vi "induction-furnace-control.vi"() -> ()   [LabVIEW 2019]
uses:
  <vilib>/DAQmx/read.llb/DAQmx Read (Analog 1D DBL 1Chan NSamp).vi
  <vilib>/Analysis/baseanly.llb/Mean (DBL).vi
  <vilib>/DAQmx/write.llb/DAQmx Write (Analog DBL 1Chan 1Samp).vi
  <vilib>/addons/control/pid/pid.llb/PID (DBL).vi
  <vilib>/DAQmx/create/channels.llb/DAQmx Create Channel (AO-Current-Basic).vi
  <vilib>/DAQmx/create/channels.llb/DAQmx Create Channel (AI-Current-Basic).vi
  <vilib>/DAQmx/miscellaneous.llb/DAQmx Fill In Error Info.vi
  <vilib>/addons/control/pid/NI_PID_pid.lvlib
  <vilib>/Analysis/NI_AALBase.lvlib
panel:
  out "VALVE OUTPUT":dbl
  in  "ENABLE FURNACE":bool[](array[boolean])
  in  "STOP FURNACE":bool[](array[boolean])
  in  "CLOSE VALVE":bool[](array[boolean])
  in  "PURGE FLOW":bool[](array[boolean])
  in  "Emergency":bool
  in  "ESTOP":bool
  in  "POWER OUT":dbl format="%#_13g"
  out "PYROMETER TEMP":dbl
  out "DONE":bool
  in  "ARGON OUT":dbl format="%#_13g"
  in  "MAIN STATE":T1(ring)
  out "MAIN PAGES":T2(tab)
  in  "TEST SETTINGS":bool
  in  "START TEST CYCLE":bool
  in  "START ARGON PURGE CYCLE":bool
  out "TIME TILL PURGE CYCLE FINISHES":dbl
  in  "START HEATING CYCLE":bool
  out "CURRENT RAMP UP POWER LEVEL":string
  out "PYROMETER TEMP RAMP UP":dbl
  out "FINAL TEMPERATURE GOAL (C)":dbl
  out "CURRENT SET POINT (C)":dbl
  out "CURRENT TEMPERATURE (C)":dbl
  out "POWER LEVEL OUTPUT (%)":dbl
  out "TEMPERATURE OVER TIME":cluster{dbl[], dbl[]}[](graph)
  out "CURRENT RAMP DOWN POWER LEVEL":string
  in  "END PROGRAM":bool
  in  "RESET PROGRAM":bool
  in  "GO BACK":bool
  in  "HOLD TIME (min)":dbl
  in  "PURGE TIMER TIME (min)":dbl
  in  "PID FINAL TEMP (C)":dbl
  in  "PID CONTROL START TEMP (C)":dbl=850.0
  in  "SAVE SETTINGS":bool
  # "Once you have loaded your sample, drawn a high vacuum, and are ready to start your test press the button below"
  # "Once you have started the purge cycle on the vacuum pump, press the button below to start the argon purge flow."
  # "min"
  # "Once you are ready to start heating up the sample, press the button below"
  # "CYCLE IS NOW FINISHED, PLEASE UNPLUG THE MASS FLOW METER.\nIF YOU WANT TO START ANOTHER TEST PRESS THE RESET BUTTON BELOW. IF NOT PRESS END."
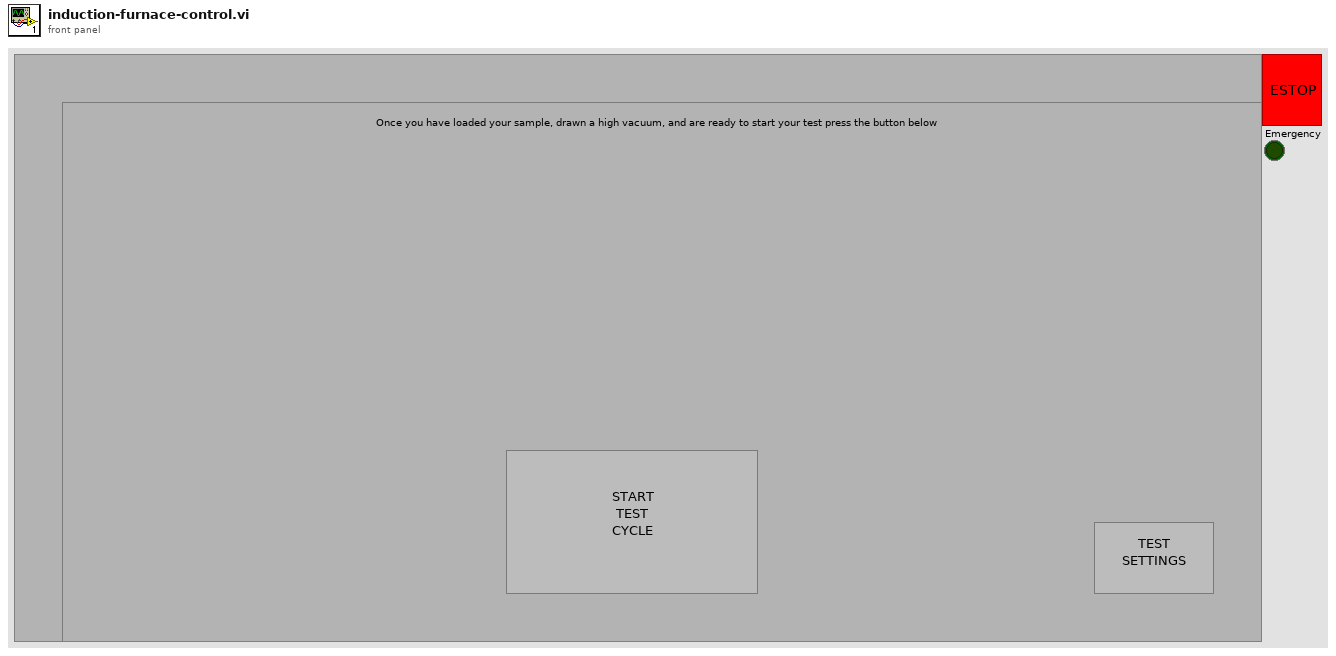
[diagram p1: front panel]
types:
  T1 = enum16{"INIT", "IDLE", "START CYCLE", "START ARGON PURGE", "ARGON TIMER", "START ARGON FLOW", "START HEATING CYCLE", "RAMP UP", "PID CONTROL", "HOLD", "PID DOWN", "RAMP DOWN", "END"}
  T2 = enum32{"START CYCLE", "START ARGON PURGE", "PURGE TIMER", "START HEATING CYCLE", "RAMP UP", "PID", "RAMP DOWN", "CYCLE FINISHED", "SETTINGS"}
  T3 = cluster{"proportional gain (Kc)":dbl, "integral time (Ti, min)":dbl, "derivative time (Td, min)":dbl}
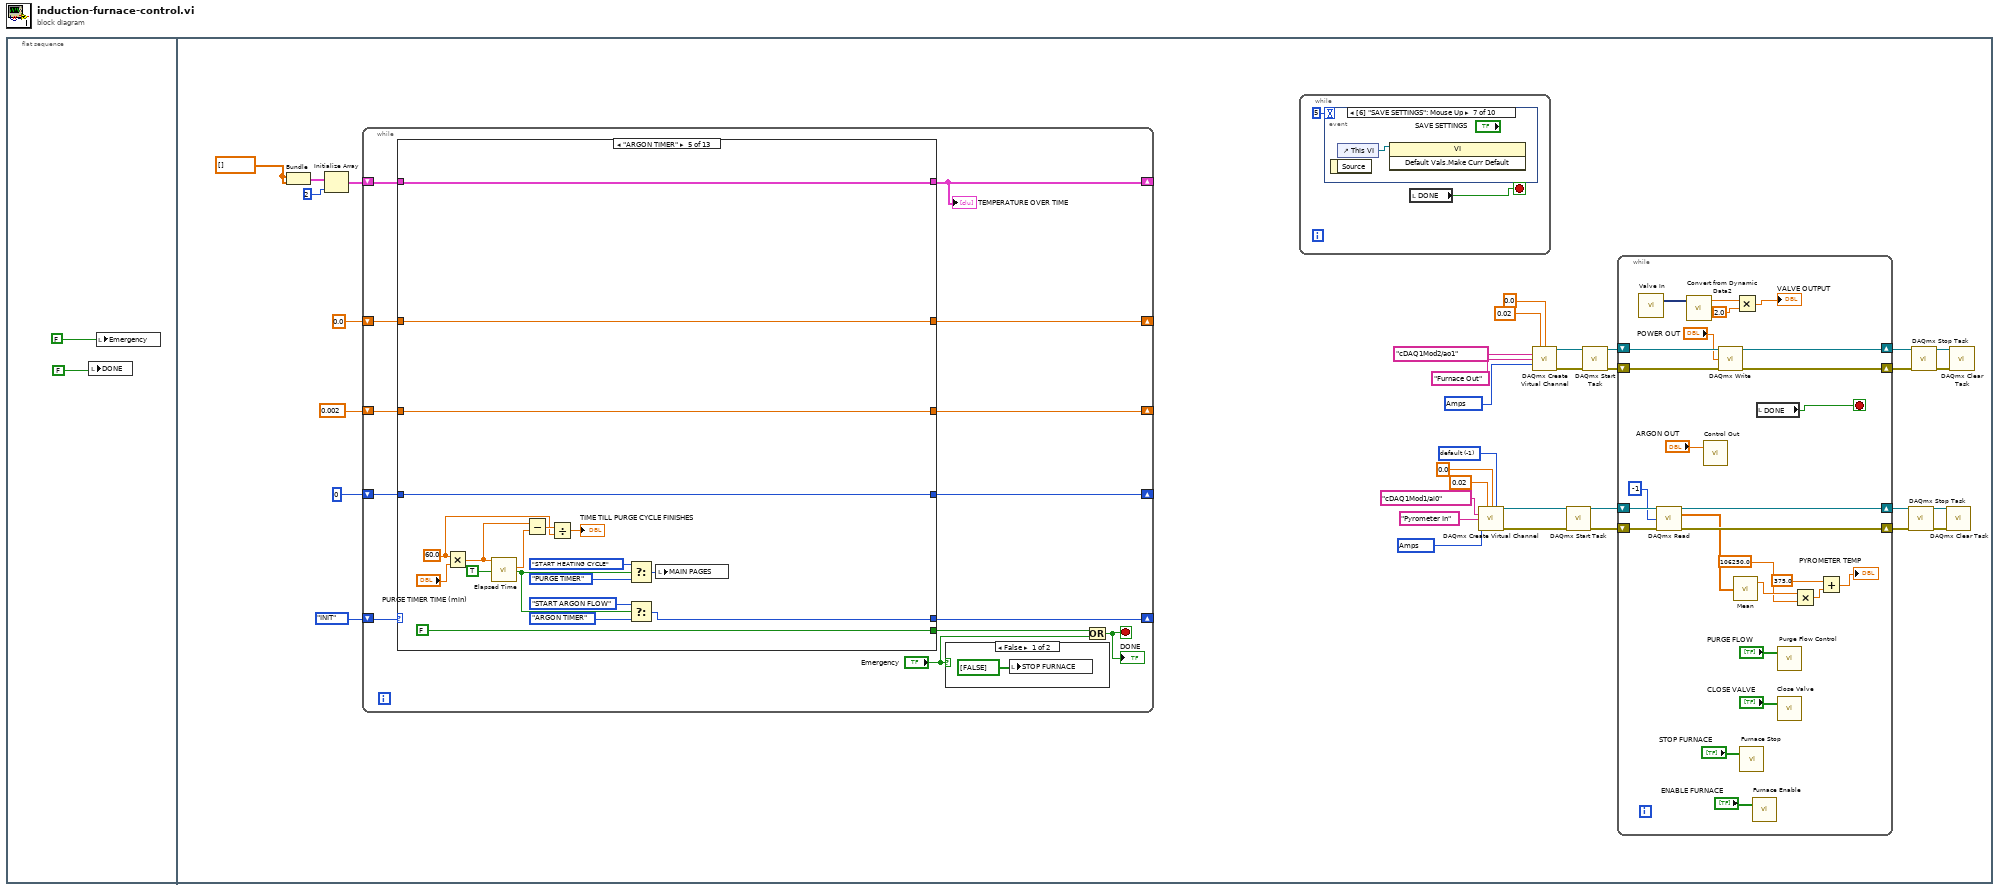
[diagram p0: block diagram]
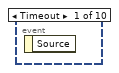
[diagram p2: hidden frame]
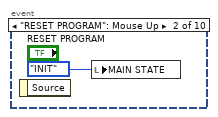
[diagram p3: hidden frame]
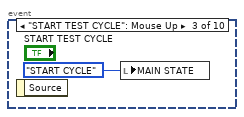
[diagram p4: hidden frame]
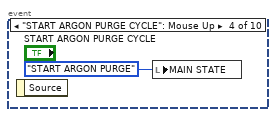
[diagram p5: hidden frame]
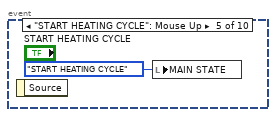
[diagram p6: hidden frame]
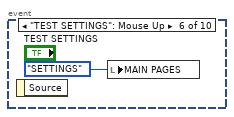
[diagram p7: hidden frame]
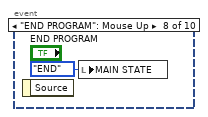
[diagram p8: hidden frame]
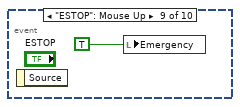
[diagram p9: hidden frame]
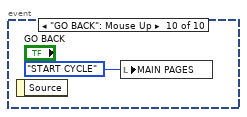
[diagram p10: hidden frame]
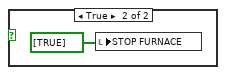
[diagram p11: hidden frame]
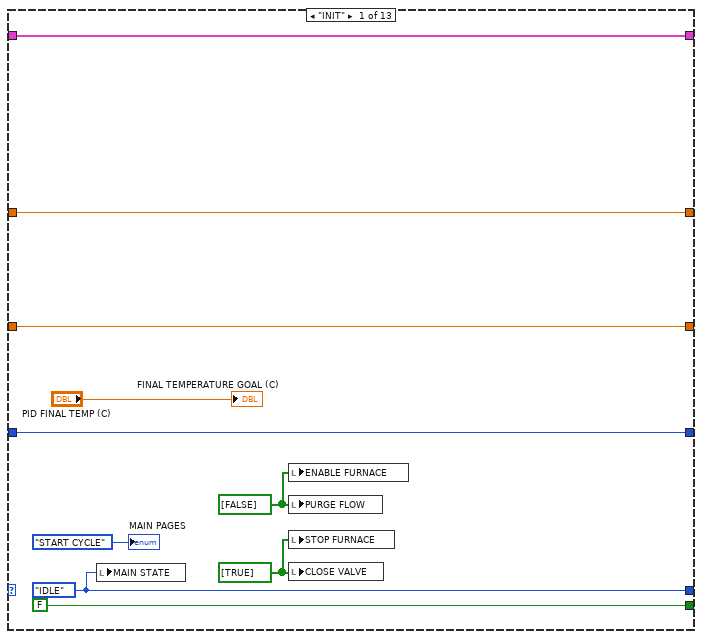
[diagram p12: hidden frame]
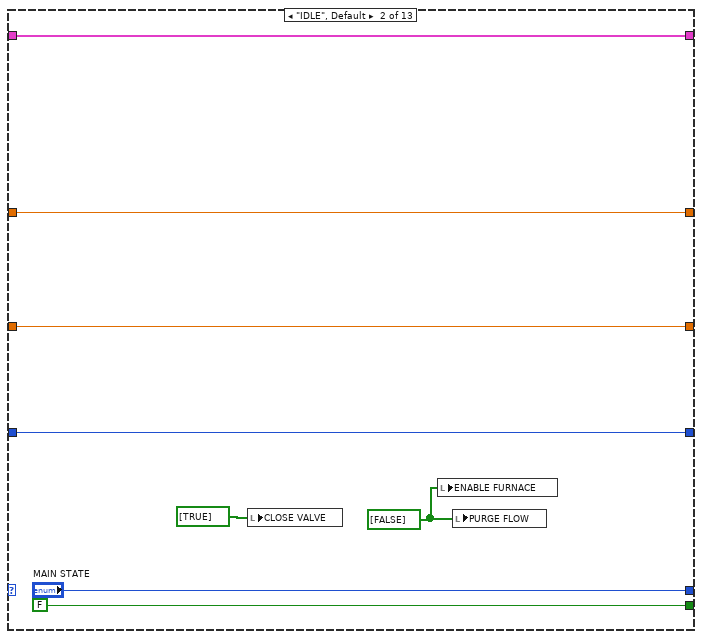
[diagram p13: hidden frame]
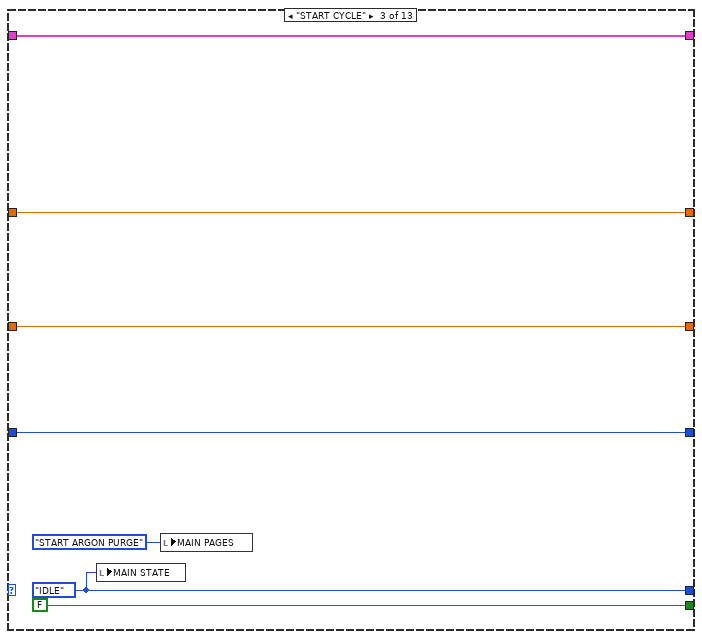
[diagram p14: hidden frame]
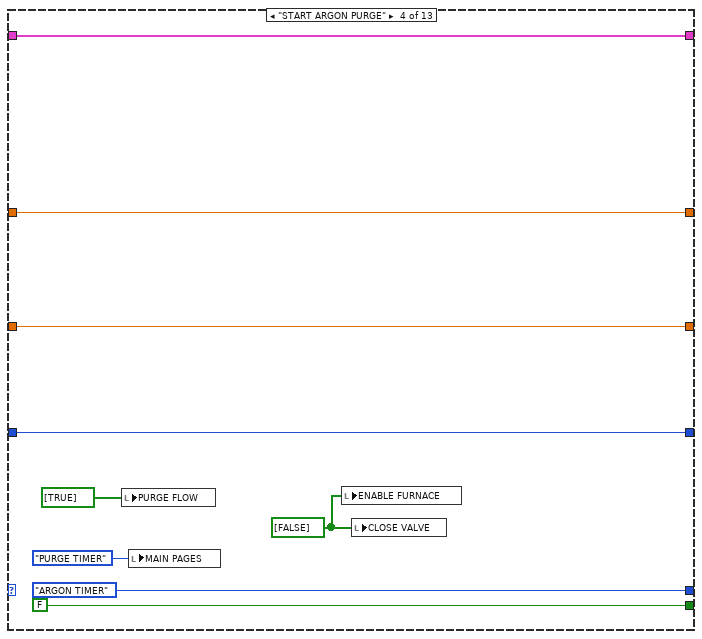
[diagram p15: hidden frame]
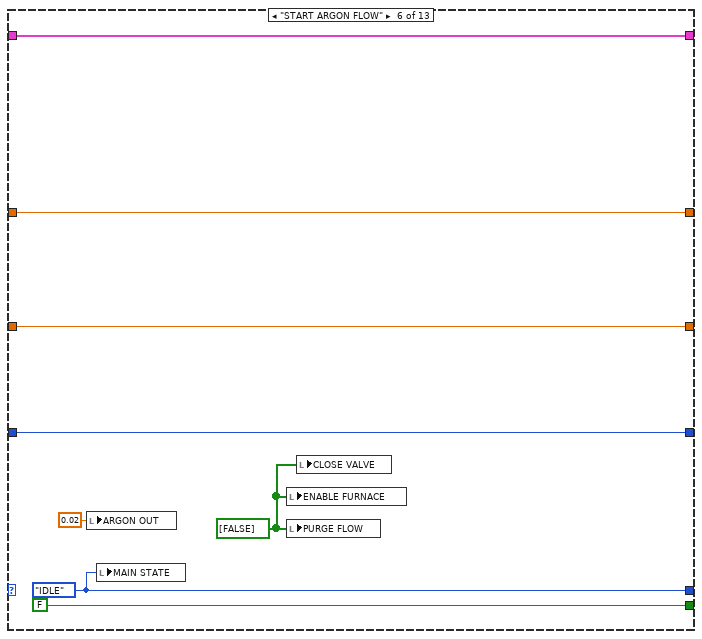
[diagram p16: hidden frame]
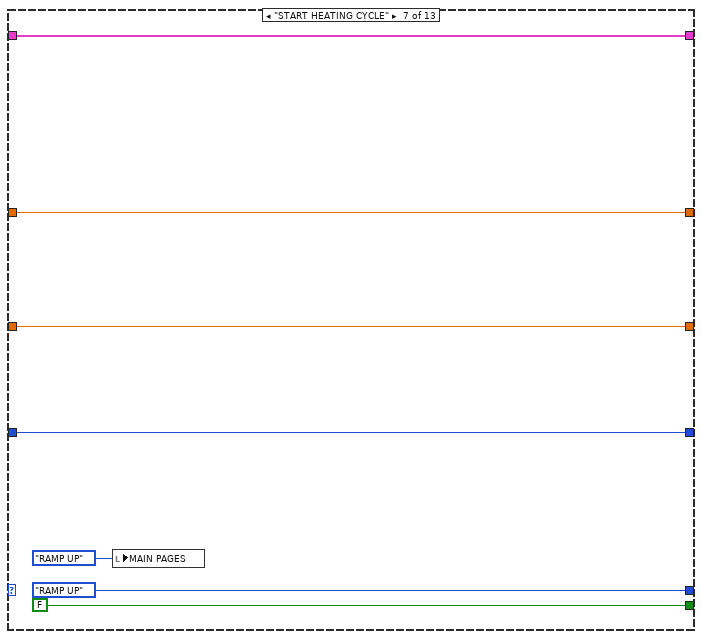
[diagram p17: hidden frame]
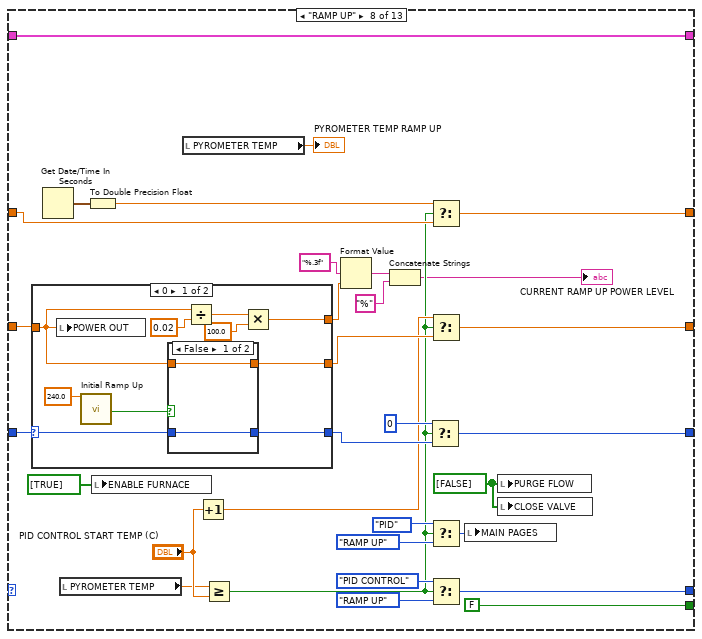
[diagram p18: hidden frame]
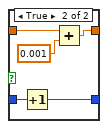
[diagram p19: hidden frame]
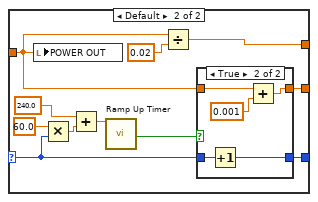
[diagram p20: hidden frame]
diagram:
  n1 = flat-sequence {
    frame #0 {
      n2 = local write "DONE"(FALSE) -> ()
      n3 = local write "Emergency"(FALSE) -> ()
    }
    frame #1 {
      w11 = -1 items=["default"=-1, "RSE"=10083, "NRSE"=10078, "Differential"=10106, "Pseudodifferential"=12529] ("input terminal configuration")
      w12 = 10342 items=["Amps"=10342, "From Custom Scale"=10065] ("units")
      w17 = 10342 items=["Amps"=10342, "From Custom Scale"=10065] ("units")
      w34 = dbl[] []
      n4 = Bundle(w34, w34) -> (w36:cluster{dbl[], dbl[]})  [unwired: 1 in]
      n5 = Initialize Array(w36, 2 ("dimension size")) -> (w33:cluster{dbl[], dbl[]}[])
      n6 = while {
        shift-right: [w86] -> _
        shift-left: T1."INIT" -> [w87]
        shift-right: [w76] -> _
        shift-left: w33 -> [w83]
        shift-right: [w81] -> _
        shift-left: 0.002 ("Ramp Power") -> [w82]
        shift-right: [w79] -> _
        shift-left: 0 ("Ramp Up Counter") -> [w80]
        shift-right: [w77] -> _
        shift-left: 0.0 ("PID Start Time") -> [w78]
        stop <- w84 stop-if-true
        n7 = case shown="\"ARGON TIMER\"" w87 {
          tunnel: [w99 "MAIN STATE" w112 T1."ARGON TIMER" ("MAIN STATE") w133 w148 T1."RAMP UP" w183 w246 w271 w315 w381 T1."END" ("MAIN STATE")] -> w86
          tunnel: [FALSE FALSE FALSE FALSE FALSE FALSE FALSE FALSE FALSE FALSE FALSE FALSE TRUE] -> w85
          tunnel: w83 -> [w94 w105 w111 w119 w128 w147 w154 w180 w239 w292 w322 w377 w396]
          tunnel: [w94 w105 w111 w119 w128 w147 w154 w180 w225 w291 w319 w377 w396] -> w76
          tunnel: w82 -> [w92 w104 w110 w117 w126 w146 w153 w178 w256 w276 w345 w376 w392]
          tunnel: [w92 w104 w110 w117 w126 w146 w153 w171 w229 w276 w311 w366 w392] -> w81
          tunnel: w80 -> [w91 w103 w109 w118 w125 w145 w152 w176 w224 w277 w318 w371 w391]
          tunnel: [w91 w103 w109 w118 w125 w145 w152 w174 w224 w277 w318 w371 w391] -> w79
          tunnel: w78 -> [w90 w102 w108 w116 w124 w144 w151 w167 w242 w290 w321 w365 _]
          tunnel: [w90 w102 w108 w116 w124 w144 w151 w164 w242 w290 w321 w365 0.0 ("PID Start Time")] -> w77
          frame "INIT" {
            w95 = bool[] [FALSE] ("CLOSE VALVE")
            w96 = bool[] [TRUE] ("CLOSE VALVE")
            w99 = T1."IDLE" ("MAIN STATE")
            n8 = local write "MAIN STATE"(w99) -> ()
            n9 = local write "ENABLE FURNACE"(w95) -> ()
            n10 = local write "PURGE FLOW"(w95) -> ()
            n11 = local write "STOP FURNACE"(w96) -> ()
            n12 = local write "CLOSE VALVE"(w96) -> ()
            "MAIN PAGES" <- T2."START CYCLE" ("MAIN PAGES")
            "FINAL TEMPERATURE GOAL (C)" <- "PID FINAL TEMP (C)"
          }
          frame "IDLE", Default {
            w100 = bool[] [FALSE] ("CLOSE VALVE")
            n13 = local write "CLOSE VALVE"(bool[] [TRUE] ("CLOSE VALVE")) -> ()
            n14 = local write "ENABLE FURNACE"(w100) -> ()
            n15 = local write "PURGE FLOW"(w100) -> ()
          }
          frame "START CYCLE" {
            w112 = T1."IDLE" ("MAIN STATE")
            n16 = local write "MAIN STATE"(w112) -> ()
            n17 = local write "MAIN PAGES"(T2."START ARGON PURGE" ("MAIN PAGES")) -> ()
          }
          frame "START ARGON PURGE" {
            w115 = bool[] [FALSE] ("CLOSE VALVE")
            n18 = local write "PURGE FLOW"(bool[] [TRUE] ("CLOSE VALVE")) -> ()
            n19 = local write "MAIN PAGES"(T2."PURGE TIMER" ("MAIN PAGES")) -> ()
            n20 = local write "ENABLE FURNACE"(w115) -> ()
            n21 = local write "CLOSE VALVE"(w115) -> ()
          }
          frame "ARGON TIMER" {
            w138 = 60.0 ("y")
            n22 = Multiply(x=w138, y="PURGE TIMER TIME (min)") -> (x*y=w142:dbl)
            n23 = call "Elapsed Time"("Time Target (s)"=w142, "Auto Reset"=TRUE ("Reset")) -> ("Elapsed Time (s)"=w141:dbl, "Time has Elapsed"=w132:bool)  [unwired: 10 in, 6 out]
            n24 = Subtract(x=w142, y=w141) -> (x-y=w139:dbl)
            n25 = Divide(x=w139, y=w138) -> (x/y=→"TIME TILL PURGE CYCLE FINISHES":dbl)
            n26 = Select(t=T2."START HEATING CYCLE" ("MAIN PAGES"), s=w132, f=T2."PURGE TIMER" ("MAIN PAGES")) -> (s? t:f=w131:T2)
            n27 = Select(t=T1."START ARGON FLOW", s=w132, f=T1."ARGON TIMER") -> (s? t:f=w133:T1)
            n28 = local write "MAIN PAGES"(w131) -> ()
          }
          frame "START ARGON FLOW" {
            w143 = bool[] [FALSE] ("CLOSE VALVE")
            w148 = T1."IDLE" ("MAIN STATE")
            n29 = local write "ARGON OUT"(0.02 ("CONTROL OUT")) -> ()
            n30 = local write "MAIN STATE"(w148) -> ()
            n31 = local write "ENABLE FURNACE"(w143) -> ()
            n32 = local write "PURGE FLOW"(w143) -> ()
            n33 = local write "CLOSE VALVE"(w143) -> ()
          }
          frame "START HEATING CYCLE" {
            n34 = local write "MAIN PAGES"(T2."RAMP UP" ("MAIN PAGES")) -> ()
          }
          frame "RAMP UP" {
            w182 = bool[] [FALSE] ("CLOSE VALVE")
            n35 = case shown="0" w176 {
              selector: w176 -> [w196 w208]
              tunnel: [w190 w214] -> w177
              tunnel: w178 -> [w195 w213]
              tunnel: [w193 w207] -> w172
              tunnel: [w192 w206] -> w173
              frame 0 {
                n36 = local write "POWER OUT"(w195) -> ()
                n37 = call "Initial Ramp Up"("Time Target (s)"=240.0) -> ("Time has Elapsed"=w198:bool)  [unwired: 11 in, 7 out]
                n38 = case shown="False" w198 {
                  tunnel: w196 -> [w199 w205]
                  tunnel: w195 -> [w200 w204]
                  tunnel: [w200 w202] -> w193
                  tunnel: [w199 w201] -> w192
                  frame False {
                  }
                  frame True {
                    n39 = Increment(x=w205) -> (x+1=w201:i32)
                    n40 = Add(x=w204, y=0.001) -> (x+y=w202:dbl)
                  }
                }
                n41 = Divide(x=w195, y=0.02) -> (x/y=w191:dbl)
                n42 = Multiply(x=w191, y=100.0) -> (x*y=w190:dbl)
              }
              frame Default {
                n43 = local write "POWER OUT"(w213) -> ()
                n44 = Multiply(x=60.0 ("Time Target (s)"), y=w208) -> (x*y=w211:dbl)
                n45 = Add(x=240.0 ("Time Target (s)"), y=w211) -> (x+y=w210:dbl)
                n46 = call "Ramp Up Timer"("Time Target (s)"=w210) -> ("Time has Elapsed"=w216:bool)  [unwired: 11 in, 7 out]
                n47 = Divide(x=w213, y=0.02) -> (x/y=w214:dbl)
                n48 = case shown="True" w216 {
                  tunnel: w208 -> [w218 w223]
                  tunnel: w213 -> [w217 w222]
                  tunnel: [w217 w220] -> w207
                  tunnel: [w218 w219] -> w206
                  frame False {
                  }
                  frame True {
                    n49 = Increment(x=w223) -> (x+1=w219:i32)
                    n50 = Add(x=w222, y=0.001) -> (x+y=w220:dbl)
                  }
                }
              }
            }
            n51 = Get Date/Time In Seconds() -> (seconds since 1Jan1904=w170:timestamp)
            n52 = local read "PYROMETER TEMP"() -> (w162:dbl)
            n53 = To Double Precision Float(number=w170) -> (double precision float=w166:dbl)
            n54 = local write "ENABLE FURNACE"(bool[] [TRUE] ("CLOSE VALVE")) -> ()
            n55 = local read "PYROMETER TEMP"() -> (→"PYROMETER TEMP RAMP UP":dbl)
            n56 = Increment(x="PID CONTROL START TEMP (C)") -> (x+1=w169:dbl)
            n57 = Greater Or Equal?(x=w162, y="PID CONTROL START TEMP (C)") -> (x >= y?=w165:bool)
            n58 = Format Value(format string="%.3f", value (0)=w177) -> (output string=w161:string)  [unwired: 1 in]
            n59 = Concatenate Strings(w161, "%" ("format string")) -> (→"CURRENT RAMP UP POWER LEVEL":string)
            n60 = Select(t=0 ("Ramp Up Counter"), s=w165, f=w173) -> (s? t:f=w174:i32)
            n61 = Select(t=w166, s=w165, f=w167) -> (s? t:f=w164:dbl)
            n62 = Select(t=w169, s=w165, f=w172) -> (s? t:f=w171:dbl)
            n63 = Select(t=T2."PID" ("MAIN PAGES"), s=w165, f=T2."RAMP UP" ("MAIN PAGES")) -> (s? t:f=w188:T2)
            n64 = Select(t=T1."PID CONTROL", s=w165, f=T1."RAMP UP") -> (s? t:f=w183:T1)
            n65 = local write "MAIN PAGES"(w188) -> ()
            n66 = local write "PURGE FLOW"(w182) -> ()
            n67 = local write "CLOSE VALVE"(w182) -> ()
          }
          frame "PID CONTROL" {
            w262 = bool[] [FALSE] ("CLOSE VALVE")
            n68 = Get Date/Time In Seconds() -> (seconds since 1Jan1904=w260:timestamp)
            n69 = local read "PID FINAL TEMP (C)"() -> (w245:dbl)
            n70 = call "Rate Delay"("Time Target (s)"=6.0) -> ("Time has Elapsed"=w257:bool)  [unwired: 11 in, 7 out]
            n71 = To Double Precision Float(number=w260) -> (double precision float=w259:dbl)
            n72 = Subtract(x=w259, y=w242) -> (x-y=w235:dbl)
            n73 = local write "MAIN PAGES"(T2."PID" ("MAIN PAGES")) -> ()
            n74 = local write "PURGE FLOW"(w262) -> ()
            n75 = local write "CLOSE VALVE"(w262) -> ()
            n76 = local write "ENABLE FURNACE"(bool[] [TRUE] ("CLOSE VALVE")) -> ()
            n77 = local read "PYROMETER TEMP"() -> (w233:dbl)
            "CURRENT TEMPERATURE (C)" <- w233
            n78 = Index Array(array=w239, index #1=0 ("index"), index #2=1 ("index")) -> (element #1=w238:cluster{dbl[], dbl[]}, element #2=w237:cluster{dbl[], dbl[]})
            n79 = case shown="True" w257 {
              tunnel: w256 -> [w265 w267]
              tunnel: [w265 w268] -> w229
              tunnel: w245 -> [_ w270]
              tunnel: [FALSE w266] -> w244
              frame False {
              }
              frame True {
                n80 = Increment(x=w267) -> (x+1=w269:dbl)
                n81 = Equal?(x=w267, y=w270) -> (x = y?=w266:bool)
                n82 = Select(t=w267, s=w266, f=w269) -> (s? t:f=w268:dbl)
              }
            }
            "CURRENT SET POINT (C)" <- w229
            n83 = Unbundle(w238) -> (w236:dbl[], w232:dbl[])
            n84 = Unbundle(w237) -> (w230:dbl[])  [unwired: 1 out]
            n85 = Select(t=T1."HOLD", s=w244, f=T1."PID CONTROL") -> (s? t:f=w246:T1)
            n86 = Build Array (concatenate)(w236, w235) -> (w234:dbl[])
            n87 = Build Array (concatenate)(w232, w233) -> (w231:dbl[])
            n88 = Build Array (concatenate)(w230, w229) -> (w228:dbl[])
            n89 = Bundle(cluster=w238, w234, w231) -> (w227:cluster{dbl[], dbl[]})
            n90 = Bundle(cluster=w237, w234, w228) -> (w226:cluster{dbl[], dbl[]})
            n91 = call-poly <vilib>:"PID.vi"("reinitialize? (F)"=FALSE, "output range"=cluster{"output high":dbl, "output low":dbl} {"output high"=0.008, "output low"=0.002}, "dt (s)"=0.06, "PID gains"=T3 {"proportional gain (Kc)"=5e-05, "integral time (Ti, min)"=1.5, "derivative time (Td, min)"=0.0}, "process variable"=w233, "setpoint"=w229) -> ("output"=w243:dbl)  [unwired: 4 in, 1 out]
            n92 = local write "POWER OUT"(w243) -> ()
            n93 = Build Array(w227, w226) -> (w225:cluster{dbl[], dbl[]}[])
            n94 = Multiply(x=5000.0 ("y"), y=w243) -> (x*y=→"POWER LEVEL OUTPUT (%)":dbl)
          }
          frame "HOLD" {
            w308 = bool[] [FALSE] ("CLOSE VALVE")
            n95 = local read "PYROMETER TEMP"() -> (w281:dbl)
            n96 = Get Date/Time In Seconds() -> (seconds since 1Jan1904=w306:timestamp)
            n97 = Multiply(x="HOLD TIME (min)", y=60.0 ("Time Target (s)")) -> (x*y=w284:dbl)
            n98 = To Double Precision Float(number=w306) -> (double precision float=w305:dbl)
            n99 = call "Hold Delay"("Time Target (s)"=w284) -> ("Time has Elapsed"=w272:bool)  [unwired: 11 in, 7 out]
            n100 = Index Array(array=w292, index #1=0 ("index"), index #2=1 ("index")) -> (element #1=w302:cluster{dbl[], dbl[]}, element #2=w283:cluster{dbl[], dbl[]})
            n101 = Subtract(x=w305, y=w290) -> (x-y=w300:dbl)
            n102 = Unbundle(w302) -> (w301:dbl[], w298:dbl[])
            n103 = Unbundle(w283) -> (w296:dbl[])  [unwired: 1 out]
            n104 = local write "MAIN PAGES"(T2."PID" ("MAIN PAGES")) -> ()
            n105 = local write "PURGE FLOW"(w308) -> ()
            n106 = local write "CLOSE VALVE"(w308) -> ()
            n107 = local write "ENABLE FURNACE"(bool[] [TRUE] ("CLOSE VALVE")) -> ()
            n108 = Select(t=T1."PID DOWN", s=w272, f=T1."HOLD") -> (s? t:f=w271:T1)
            n109 = local write "CURRENT SET POINT (C)"(w276) -> ()
            n110 = local write "CURRENT TEMPERATURE (C)"(w281) -> ()
            n111 = Build Array (concatenate)(w301, w300) -> (w299:dbl[])
            n112 = Build Array (concatenate)(w298, w281) -> (w297:dbl[])
            n113 = Build Array (concatenate)(w296, w276) -> (w295:dbl[])
            n114 = Bundle(cluster=w302, w299, w297) -> (w294:cluster{dbl[], dbl[]})
            n115 = Bundle(cluster=w283, w299, w295) -> (w293:cluster{dbl[], dbl[]})
            n116 = call-poly <vilib>:"PID.vi"("reinitialize? (F)"=FALSE, "output range"=cluster{"output high":dbl, "output low":dbl} {"output high"=0.02, "output low"=0.002}, "dt (s)"=0.06, "PID gains"=T3 {"proportional gain (Kc)"=5e-05, "integral time (Ti, min)"=1.5, "derivative time (Td, min)"=0.0}, "process variable"=w281, "setpoint"=w276) -> ("output"=w278:dbl)  [unwired: 4 in, 1 out]
            n117 = local write "POWER OUT"(w278) -> ()
            n118 = Build Array(w294, w293) -> (w291:cluster{dbl[], dbl[]}[])
            n119 = Multiply(x=5000.0 ("y"), y=w278) -> (x*y=w282:dbl)
            n120 = local write "POWER LEVEL OUTPUT (%)"(w282) -> ()
          }
          frame "PID DOWN" {
            w349 = bool[] [FALSE] ("CLOSE VALVE")
            n121 = local read "PID CONTROL START TEMP (C)"() -> (w344:dbl)
            n122 = local read "PID CONTROL START TEMP (C)"() -> (w350:dbl)
            n123 = local read "PYROMETER TEMP"() -> (w320:dbl)
            n124 = call "Rate Delay Down"("Time Target (s)"=12.0) -> ("Time has Elapsed"=w347:bool)  [unwired: 11 in, 7 out]
            n125 = local write "MAIN PAGES"(T2."PID" ("MAIN PAGES")) -> ()
            n126 = local write "ENABLE FURNACE"(bool[] [TRUE] ("CLOSE VALVE")) -> ()
            n127 = local write "PURGE FLOW"(w349) -> ()
            n128 = local write "CLOSE VALVE"(w349) -> ()
            n129 = Get Date/Time In Seconds() -> (seconds since 1Jan1904=w337:timestamp)
            n130 = To Double Precision Float(number=w337) -> (double precision float=w336:dbl)
            n131 = local write "FINAL TEMPERATURE GOAL (C)"(w350) -> ()
            n132 = case shown="True" w347 {
              tunnel: w345 -> [w353 w356]
              tunnel: [w353 w357] -> w312
              tunnel: [FALSE w355] -> w313
              tunnel: w344 -> [_ w354]
              frame False {
              }
              frame True {
                n133 = Decrement(x=w356) -> (x-1=w358:dbl)
                n134 = Equal?(x=w356, y=w354) -> (x = y?=w355:bool)
                n135 = Select(t=w356, s=w355, f=w358) -> (s? t:f=w357:dbl)
              }
            }
            n136 = Index Array(array=w322, index #1=0 ("index"), index #2=1 ("index")) -> (element #1=w335:cluster{dbl[], dbl[]}, element #2=w325:cluster{dbl[], dbl[]})
            n137 = Subtract(x=w336, y=w321) -> (x-y=w333:dbl)
            n138 = Unbundle(w335) -> (w334:dbl[], w331:dbl[])
            n139 = Unbundle(w325) -> (w329:dbl[])  [unwired: 1 out]
            n140 = Build Array (concatenate)(w334, w333) -> (w332:dbl[])
            n141 = Build Array (concatenate)(w331, w320) -> (w330:dbl[])
            n142 = Build Array (concatenate)(w329, w312) -> (w328:dbl[])
            n143 = local write "CURRENT SET POINT (C)"(w312) -> ()
            n144 = local write "CURRENT TEMPERATURE (C)"(w320) -> ()
            n145 = Select(t=T1."RAMP DOWN" ("MAIN STATE"), s=w313, f=T1."PID DOWN" ("MAIN STATE")) -> (s? t:f=w315:T1)
            n146 = Bundle(cluster=w335, w332, w330) -> (w327:cluster{dbl[], dbl[]})
            n147 = Bundle(cluster=w325, w332, w328) -> (w326:cluster{dbl[], dbl[]})
            n148 = call-poly <vilib>:"PID.vi"("reinitialize? (F)"=FALSE, "output range"=cluster{"output high":dbl, "output low":dbl} {"output high"=0.008, "output low"=0.002}, "dt (s)"=0.06, "PID gains"=T3 {"proportional gain (Kc)"=5e-05, "integral time (Ti, min)"=1.5, "derivative time (Td, min)"=0.0}, "process variable"=w320, "setpoint"=w312) -> ("output"=w310:dbl)  [unwired: 4 in, 1 out]
            n149 = local write "POWER OUT"(w310) -> ()
            n150 = Build Array(w327, w326) -> (w319:cluster{dbl[], dbl[]}[])
            n151 = Multiply(x=5000.0 ("y"), y=w310) -> (x*y=w343:dbl)
            n152 = local write "POWER LEVEL OUTPUT (%)"(w343) -> ()
            n153 = Select(t=w310, s=w313, f=w312) -> (s? t:f=w311:dbl)
          }
          frame "RAMP DOWN" {
            w379 = bool[] [FALSE] ("CLOSE VALVE")
            w380 = T1."IDLE"
            n154 = local write "POWER OUT"(w376) -> ()
            n155 = local write "ENABLE FURNACE"(bool[] [TRUE] ("CLOSE VALVE")) -> ()
            n156 = local write "PURGE FLOW"(w379) -> ()
            n157 = local write "CLOSE VALVE"(w379) -> ()
            n158 = call "Ramp Down Timer"("Time Target (s)"=90.0) -> ("Time has Elapsed"=w375:bool)  [unwired: 11 in, 7 out]
            n159 = Divide(x=w376, y=0.02) -> (x/y=w364:dbl)
            n160 = Multiply(x=w364, y=100.0) -> (x*y=w362:dbl)
            n161 = case shown="True" w375 {
              tunnel: w376 -> [w387 w390]
              tunnel: [w387 w388] -> w368
              frame False {
              }
              frame True {
                n162 = Subtract(x=w390, y=0.001) -> (x-y=w388:dbl)
              }
            }
            n163 = Format Value(format string="%.3f", value (0)=w362) -> (output string=w361:string)  [unwired: 1 in]
            n164 = Concatenate Strings(w361, "%" ("string")) -> (→"CURRENT RAMP DOWN POWER LEVEL":string)
            n165 = Less Or Equal?(x=w368, y=0.002) -> (x <= y?=w369:bool)
            n166 = Select(t=0.0, s=w369, f=w368) -> (s? t:f=w366:dbl)
            n167 = Select(t=w380, s=w369, f=T1."RAMP DOWN") -> (s? t:f=w381:T1)
            n168 = Select(t=T2."CYCLE FINISHED" ("MAIN PAGES"), s=w369, f=T2."RAMP DOWN" ("MAIN PAGES")) -> (s? t:f=w385:T2)
            n169 = local write "MAIN PAGES"(w385) -> ()
            n170 = local write "MAIN STATE"(w380) -> ()
          }
          frame "END" {
            w395 = bool[] [FALSE] ("CLOSE VALVE")
            n171 = local write "ENABLE FURNACE"(w395) -> ()
            n172 = local write "PURGE FLOW"(w395) -> ()
            n173 = local write "CLOSE VALVE"(bool[] [TRUE] ("CLOSE VALVE")) -> ()
          }
        }
        "TEMPERATURE OVER TIME" <- w76
        n174 = case shown="False" "Emergency" {
          frame False {
            n175 = local write "STOP FURNACE"(bool[] [FALSE] ("CLOSE VALVE")) -> ()
          }
          frame True {
            n176 = local write "STOP FURNACE"(bool[] [TRUE] ("CLOSE VALVE")) -> ()
          }
        }
        n177 = Or(x=w85, y="Emergency") -> (x .or. y?=w84:bool)
        "DONE" <- w84
      }
      n178 = while {
        stop <- w64 stop-if-true
        n179 = event shown="[6] \"SAVE SETTINGS\": Mouse Up" {
          selector: _ -> [_ _ _ _ _ _ _ _ _ _]
          dyn-events: _ -> [_ _ _ _ _ _ _ _ _ _]
          timeout: 5 -> [_ _ _ _ _ _ _ _ _ _]
          event Timeout {
            n180 = event-data() -> ()  [unwired: 1 in, 1 out]
          }
          event "RESET PROGRAM": Mouse Up {
            n181 = event-data() -> ()  [unwired: 1 in, 1 out]
            n182 = local write "MAIN STATE"(T1."INIT" ("MAIN STATE")) -> ()
          }
          event "START TEST CYCLE": Mouse Up {
            n183 = event-data() -> ()  [unwired: 1 in, 1 out]
            n184 = local write "MAIN STATE"(T1."START CYCLE" ("MAIN STATE")) -> ()
          }
          event "START ARGON PURGE CYCLE": Mouse Up {
            n185 = event-data() -> ()  [unwired: 1 in, 1 out]
            n186 = local write "MAIN STATE"(T1."START ARGON PURGE" ("MAIN STATE")) -> ()
          }
          event "START HEATING CYCLE": Mouse Up {
            n187 = event-data() -> ()  [unwired: 1 in, 1 out]
            n188 = local write "MAIN STATE"(T1."START HEATING CYCLE" ("MAIN STATE")) -> ()
          }
          event "TEST SETTINGS": Mouse Up {
            n189 = event-data() -> ()  [unwired: 1 in, 1 out]
            n190 = local write "MAIN PAGES"(T2."SETTINGS" ("MAIN PAGES")) -> ()
          }
          event "SAVE SETTINGS": Mouse Up {
            n191 = event-data() -> ()  [unwired: 1 in, 1 out]
            n192 = control-ref of="This VI"() -> (w71:refnum<vi>)
            n193 = invoke class="VI" method="Default Vals.Make Curr Default"(reference=w71) -> ()  [unwired: 2 in, 3 out]
          }
          event "END PROGRAM": Mouse Up {
            n194 = event-data() -> ()  [unwired: 1 in, 1 out]
            n195 = local write "MAIN STATE"(T1."END" ("MAIN STATE")) -> ()
          }
          event "ESTOP": Mouse Up {
            n196 = event-data() -> ()  [unwired: 1 in, 1 out]
            n197 = local write "Emergency"(TRUE) -> ()
          }
          event "GO BACK": Mouse Up {
            n198 = event-data() -> ()  [unwired: 1 in, 1 out]
            n199 = local write "MAIN PAGES"(T2."START CYCLE" ("MAIN PAGES")) -> ()
          }
        }
        n200 = local read "DONE"() -> (w64:bool)
      }
      n201 = call-poly <vilib>:"DAQmx Create Virtual Channel.vi"("maximum value"=0.02, "minimum value"=0.0, "input terminal configuration"=w11, "physical channels"=tag "cDAQ1Mod1/ai0", "name to assign"="Pyrometer In", "units"=w12) -> ("task out"=w10:refnum<k21>, "error out"=w9:errorcluster)  [unwired: 8 in]
      n202 = call-poly <vilib>:"DAQmx Create Virtual Channel.vi"("maximum value"=0.02, "minimum value"=0.0, "physical channels"=tag "cDAQ1Mod2/ao1", "name to assign"="Furnace Out", "units"=w17) -> ("task out"=w25:refnum<k21>, "error out"=w24:errorcluster)  [unwired: 9 in]
      n203 = call <vilib>:"DAQmx Start Task.vi"("task/channels in"=w10, "error in"=w9) -> ("task out"=w8:refnum<k21>, "error out"=w7:errorcluster)  [unwired: 12 in]
      n204 = call <vilib>:"DAQmx Start Task.vi"("task/channels in"=w25, "error in"=w24) -> ("task out"=w23:refnum<k21>, "error out"=w22:errorcluster)  [unwired: 12 in]
      n205 = while {
        shift-right: [w54] -> w20
        shift-left: w23 -> [w57]
        shift-right: [w53] -> w19
        shift-left: w22 -> [w56]
        shift-right: [w44] -> w3
        shift-left: w7 -> [w51]
        shift-right: [w45] -> w4
        shift-left: w8 -> [w52]
        stop <- w38 stop-if-true
        n206 = call "Valve In"() -> ("data"=w61:dynamicdata)  [unwired: 16 in, 3 out]
        n207 = call-poly <vilib>:"DAQmx Read.vi"("task/channels in"=w52, "number of samples per channel"=-1, "error in"=w51) -> ("task out"=w45:refnum<k21>, "data"=w43:dbl[], "error out"=w44:errorcluster)  [unwired: 10 in]
        n208 = call "Convert from Dynamic Data2"("Dynamic Data Type"=w61) -> ("Scalar"=w60:dbl)  [unwired: 3 in]
        n209 = call "Control Out"("data"="ARGON OUT") -> ()  [unwired: 17 in, 2 out]
        n210 = call-poly <vilib>:"DAQmx Write.vi"("task/channels in"=w57, "data"="POWER OUT", "error in"=w56) -> ("task out"=w54:refnum<k21>, "error out"=w53:errorcluster)  [unwired: 10 in, 1 out]
        n211 = call-poly <vilib>:"Mean.vi"("X"=w43) -> ("mean"=w49:dbl)  [unwired: 1 out]
        n212 = Multiply(x=w60, y=2.0) -> (x*y=→"VALVE OUTPUT":dbl)
        n213 = call "Furnace Stop"("data"="STOP FURNACE") -> ()  [unwired: 17 in, 2 out]
        n214 = call "Furnace Enable"("data"="ENABLE FURNACE") -> ()  [unwired: 17 in, 2 out]
        n215 = local read "DONE"() -> (w38:bool)
        n216 = call "Purge Flow Control"("data"="PURGE FLOW") -> ()  [unwired: 17 in, 2 out]
        n217 = call "Close Valve"("data"="CLOSE VALVE") -> ()  [unwired: 17 in, 2 out]
        n218 = Multiply(x=w49, y=106250.0) -> (x*y=w48:dbl)
        n219 = Add(x=375.0, y=w48) -> (x+y=→"PYROMETER TEMP":dbl)
      }
      n220 = call <vilib>:"DAQmx Stop Task.vi"("task/channels in"=w4, "error in"=w3) -> ("task out"=w6:refnum<k21>, "error out"=w5:errorcluster)  [unwired: 12 in]
      n221 = call <vilib>:"DAQmx Stop Task.vi"("task/channels in"=w20, "error in"=w19) -> ("task out"=w21:refnum<k21>, "error out"=w18:errorcluster)  [unwired: 12 in]
      n222 = call <vilib>:"DAQmx Clear Task.vi"("task in"=w6, "error in"=w5) -> ()  [unwired: 13 in, 1 out]
      n223 = call <vilib>:"DAQmx Clear Task.vi"("task in"=w21, "error in"=w18) -> ()  [unwired: 13 in, 1 out]
    }
  }
